vi "Set Field Ramp Rate.vi"(0 "Segment (Model 430 only)":i32=1, 1 "VISA resource name":refnum<visa-resource-name>, 2 "Upper Bound (Model 430 only)":dbl=40.0, 3 "error in":T1, 4 "Ramp Rate (kG/sec)":dbl format="%.3f") -> (5 "VISA resource name out":refnum<visa-resource-name>, 6 "error out":T1)   [LabVIEW 2019]
panel:
  out "output string":string
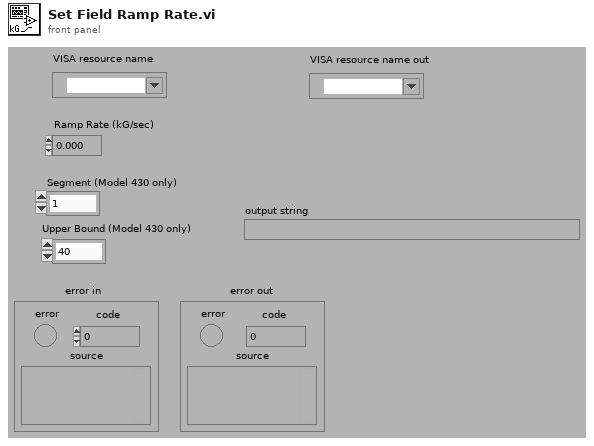
[diagram p1: front panel]
types:
  T1 = cluster{"error":bool, "code":i32, "source":string}
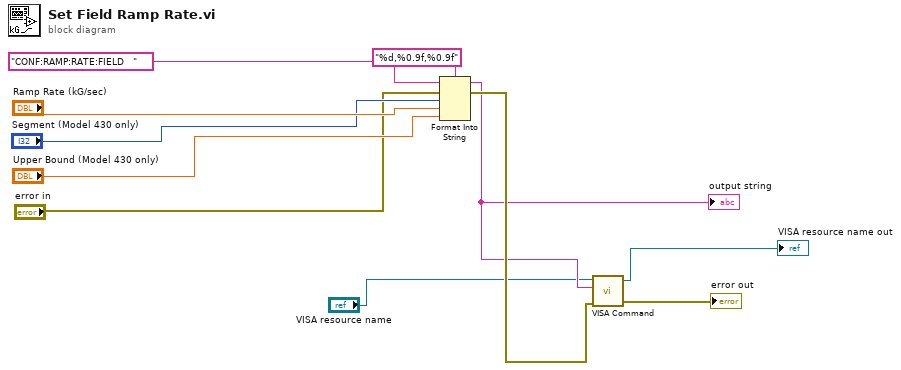
[diagram p0: block diagram]
diagram:
  n1 = Format Into String(format string="%d,%0.9f,%0.9f", initial string="CONF:RAMP:RATE:FIELD   ", error in="error in", "Segment (Model 430 only)", "Ramp Rate (kG/sec)", "Upper Bound (Model 430 only)") -> (resulting string=w5:string, error out=w6:errorcluster)
  "output string" <- w5
  n2 = call "VISA Command.vi"("error in (no error)"=w6, "Command"=w5, "VISA resource name"="VISA resource name") -> ("error out"=→"error out":errorcluster, "VISA resource name out"=→"VISA resource name out":refnum<visa-resource-name>)  [unwired: 1 in, 1 out]
